vi "CfgManager.Collection Test Launcher.vi"() -> ()   [LabVIEW 2013]
uses:
  <vilib>/LabVIEW Open Source Project/Unicity/Delimiter/Delimiters List.ctl
  source/Manager.Text/ConfigManager.Text.lvclass
  source/Manager.Text/ConfigManager.Text.lvclass/ConfigManager.Text.ctl
  source/Collection/ConfigManagerCollection.lvclass
  source/Manager/Decompose KVPs.vi
  source/Manager/Write.vi
  source/Manager/ConfigManager.lvclass
  source/Cache/ConfigManager.Cache.lvclass
  <vilib>/LabVIEW Open Source Project/Unicity/Delimiter/Delimiter.lvclass
panel:
  out "any found? 3":bool
  out "any found?":bool
  out "any found? 2":bool
  out "modified PID settings":variant
  out "all found? 3":bool
  out "all found? 2":bool
  out "all found?":bool
  out "user-defined pump config":variant
  out "default pump config":variant
  in  "default config":path
  out "merged PID settings":variant
  out "initial PID settings":variant
  out "System.Valve Keys":string[](array[string])
  out "System.Pump keys":string[](array[string])
  out "modified pump config":variant
  out "error out":errorcluster
  out "merged pump config":variant
  in  "user-defined config":path
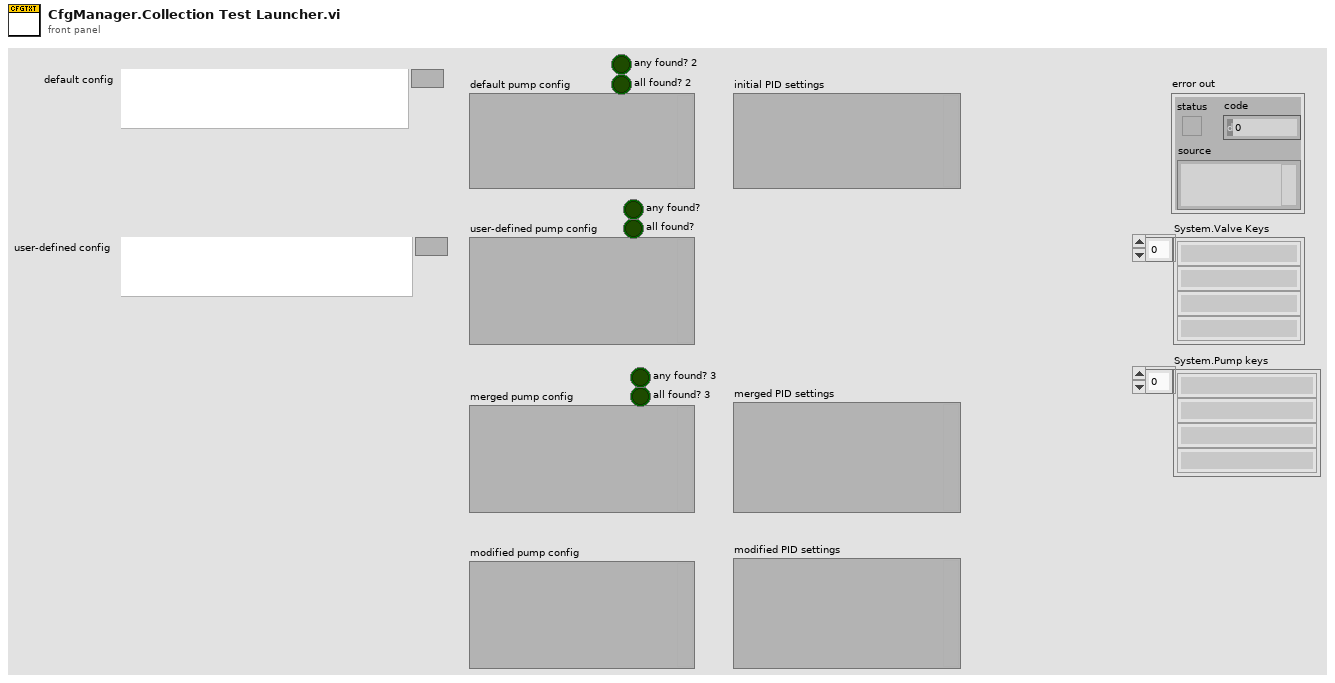
[diagram p1: front panel]
types:
  T1 = cluster{"String":string, "Numeric":dbl, "Boolean":bool}
  T2 = typedef "Delimiter.lvclass/Delimiters List.ctl" = enum16{"Default", "dot (.)", "colon (:)", "double-colon (::)", "semi-colon (;)", "underscore (_)", "double underscore (__)", "dash (-)", "double dash (--)", "backslash (\\)", "vertical bar (|)", "forward slash (/)", "chevron (>)", "double-chevron (>>)", "arrow (->)", "comma (,)", "arobas (@)", "ampersand (&)", "other"}
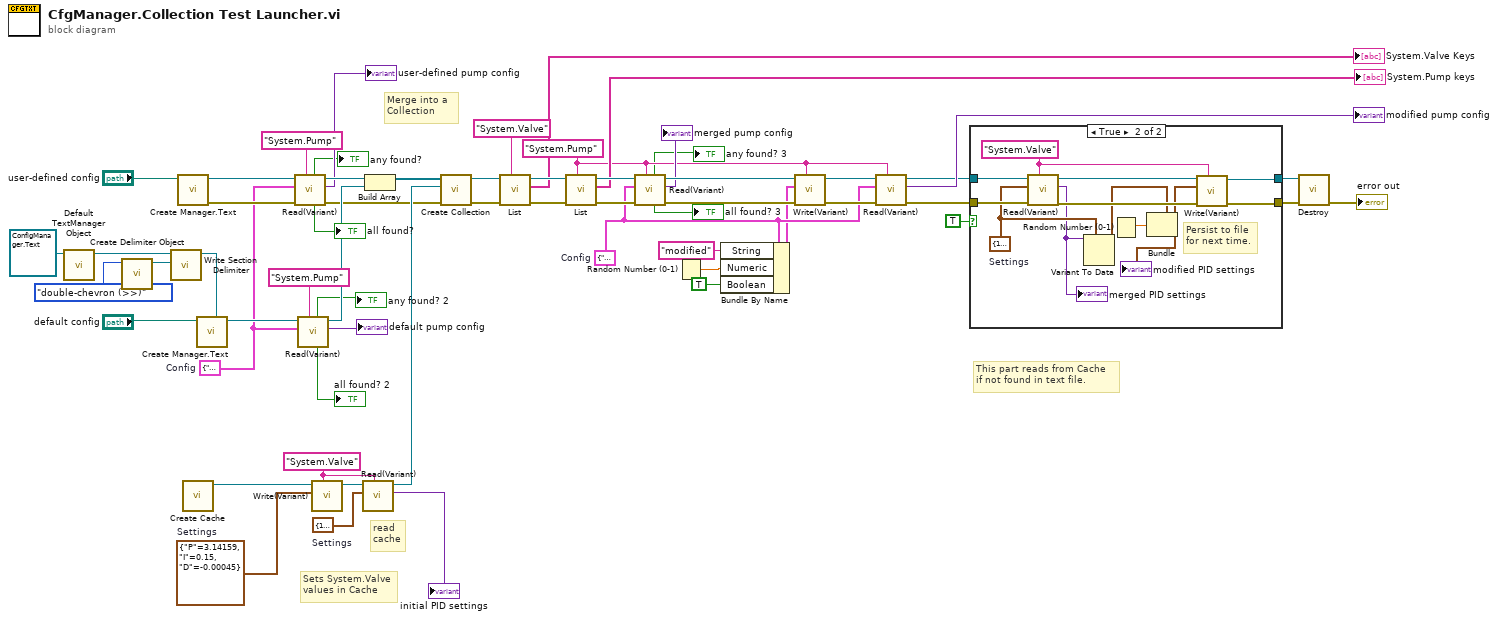
[diagram p0: block diagram]
diagram:
  w8 = T1 {"String"="", "Numeric"=0.0, "Boolean"=FALSE}  # Config
  w24 = cluster{"P":dbl, "I":dbl, "D":dbl} {"P"=1.0, "I"=0.0, "D"=0.0}  # Settings
  w40 = cluster{"P":dbl, "I":dbl, "D":dbl} {"P"=3.14159, "I"=0.15, "D"=-0.00045}  # Settings
  w25 = "System.Valve" ("Qualified Name")
  w42 = "System.Pump" ("Qualified Name")
  w41 = T1 {"String"="", "Numeric"=0.0, "Boolean"=FALSE}  # Config
  # "read\ncache"
  # "This part reads from Cache\nif not found in text file."
  # "Merge into a \nCollection"
  # "Sets System.Valve\nvalues in Cache"
  n1 = call-dynamic "Default TextManager Object.vi"("CfgManager.Text in"=refnum<class "ConfigManager.Text.lvclass"> refnum) -> ("CfgManager.Text out"=w20:refnum<class "ConfigManager.Text.lvclass">)  [unwired: 10 in]
  n2 = call <vilib>:"Create Delimiter Object.vi"("Delimiter"=Delimiters_List."double-chevron (>>)") -> ("Delimiter"=w21:refnum<class "Delimiter.lvclass">)  [unwired: 10 in]
  n3 = call "Write Section Delimiter.vi"("Section Delimiter"=w21, "ConfigManager.Text in"=w20) -> ("ConfigManager.Text out"=w19:refnum<class "ConfigManager.Text.lvclass">)  [unwired: 9 in]
  n4 = call "Create Manager.Text.vi"("filepath"="user-defined config") -> ("error out"=w13:errorcluster, "ConfigManager.Text out"=w11:refnum<class "ConfigManager.Text.lvclass">)  [unwired: 8 in, 1 out]
  n5 = call "Create Cache.vi"() -> ("ConfigManager.Cache"=w39:refnum<class "ConfigManager.Cache.lvclass">)  [unwired: 11 in]
  n6 = call "Create Manager.Text.vi"("ConfigManager.Text"=w19, "filepath"="default config") -> ("ConfigManager.Text out"=w17:refnum<class "ConfigManager.Text.lvclass">)  [unwired: 7 in, 2 out]
  n7 = call "Read(Variant).vi"("Qualified Name"="System.Pump", "error in (no error)"=w13, "Type"=w8, "ConfigManager in"=w11) -> ("error out"=w12:errorcluster, "value"=→"user-defined pump config":variant, "ConfigManager out"=w10:refnum<class "ConfigManager.Text.lvclass">, "all found?"=→"all found?":bool, "any found?"=→"any found?":bool)  [unwired: 3 in]
  n8 = call "Read(Variant).vi"("Qualified Name"="System.Pump", "Type"=w8, "ConfigManager in"=w17) -> ("value"=→"default pump config":variant, "ConfigManager out"=w16:refnum<class "ConfigManager.Text.lvclass">, "all found?"=→"all found? 2":bool, "any found?"=→"any found? 2":bool)  [unwired: 4 in, 1 out]
  n9 = call "Write(Variant).vi"("Qualified Name"=w25, "value"=w40, "ConfigManager in"=w39) -> ("ConfigManager out"=w28:refnum<class "ConfigManager.Cache.lvclass">)  [unwired: 6 in, 2 out]
  n10 = call "Read(Variant).vi"("Qualified Name"=w25, "Type"=w24, "ConfigManager in"=w28) -> ("value"=→"initial PID settings":variant, "ConfigManager out"=w27:refnum<class "ConfigManager.Cache.lvclass">)  [unwired: 4 in, 3 out]
  n11 = Build Array(w10, w16) -> (w29:refnum<class "ConfigManager.Text.lvclass">[])
  n12 = call "Create Collection.vi"("Cache"=w27, "List"=w29) -> ("ConfigManagerCollection out"=w38:refnum<class "ConfigManagerCollection.lvclass">)  [unwired: 9 in]
  n13 = call "List.vi"("Qualified Name"="System.Valve", "error in (no error)"=w12, "ConfigManager in"=w38) -> ("error out"=w36:errorcluster, "Keys"=→"System.Valve Keys":string[], "ConfigManager out"=w37:refnum<class "ConfigManagerCollection.lvclass">)  [unwired: 6 in]
  n14 = call "List.vi"("Qualified Name"=w42, "error in (no error)"=w36, "ConfigManager in"=w37) -> ("error out"=w51:errorcluster, "Keys"=→"System.Pump keys":string[], "ConfigManager out"=w50:refnum<class "ConfigManagerCollection.lvclass">)  [unwired: 6 in]
  n15 = call "Read(Variant).vi"("Qualified Name"=w42, "error in (no error)"=w51, "Type"=w41, "ConfigManager in"=w50) -> ("error out"=w55:errorcluster, "value"=→"merged pump config":variant, "ConfigManager out"=w56:refnum<class "ConfigManagerCollection.lvclass">, "all found?"=→"all found? 3":bool, "any found?"=→"any found? 3":bool)  [unwired: 3 in]
  n16 = Random Number (0-1)() -> (number: 0 to 1=w31:dbl)
  n17 = Bundle By Name(cluster=w41, "String"="modified", "Numeric"=w31, "Boolean"=TRUE) -> (w30:T1)
  n18 = call "Write(Variant).vi"("Qualified Name"=w42, "error in (no error)"=w55, "value"=w30, "ConfigManager in"=w56) -> ("error out"=w53:errorcluster, "ConfigManager out"=w54:refnum<class "ConfigManagerCollection.lvclass">)  [unwired: 5 in, 1 out]
  n19 = call "Read(Variant).vi"("Qualified Name"=w42, "error in (no error)"=w53, "Type"=w41, "ConfigManager in"=w54) -> ("error out"=w45:errorcluster, "value"=→"modified pump config":variant, "ConfigManager out"=w47:refnum<class "ConfigManagerCollection.lvclass">)  [unwired: 3 in, 2 out]
  n20 = case shown="True" TRUE {
    tunnel: w47 -> [w60 w72]
    tunnel: [w60 w67] -> w46
    tunnel: w45 -> [w59 w71]
    tunnel: [w59 w66] -> w44
    frame False {
    }
    frame True {
      w65 = cluster{"P":dbl, "I":dbl, "D":dbl} {"P"=1.0, "I"=0.0, "D"=0.0}  # Settings
      w68 = "System.Valve" ("Qualified Name")
      # "Persist to file\nfor next time."
      n21 = call "Read(Variant).vi"("Qualified Name"=w68, "error in (no error)"=w71, "Type"=w65, "ConfigManager in"=w72) -> ("error out"=w69:errorcluster, "value"=w64:variant, "ConfigManager out"=w70:refnum<class "ConfigManagerCollection.lvclass">)  [unwired: 3 in, 2 out]
      "merged PID settings" <- w64
      n22 = Variant To Data(type=w65, Variant=w64) -> (data=w62:cluster{"P":dbl, "I":dbl, "D":dbl})  [unwired: 1 in, 1 out]
      n23 = Random Number (0-1)() -> (number: 0 to 1=w63:dbl)
      n24 = Bundle(cluster=w62, "I"=w63) -> (w61:cluster{"P":dbl, "I":dbl, "D":dbl})  [unwired: 2 in]
      "modified PID settings" <- w61
      n25 = call "Write(Variant).vi"("Qualified Name"=w68, "error in (no error)"=w69, "value"=w61, "ConfigManager in"=w70) -> ("error out"=w66:errorcluster, "ConfigManager out"=w67:refnum<class "ConfigManagerCollection.lvclass">)  [unwired: 5 in, 1 out]
    }
  }
  n26 = call-dynamic "Destroy.vi"("error in (no error)"=w44, "ConfigManagerCollection in"=w46) -> ("error out"=→"error out":errorcluster)  [unwired: 8 in, 1 out]
